vi "Barker7.vi"(9 "Barker code":i16[](array[numeric])=[16384, 16384, 16384, -16384, -16384, 16384, -16384], 10 "Barker width":u16, 11 "first?":bool) -> (2 "output":i16, 3 "output valid":bool)   [LabVIEW 2017]
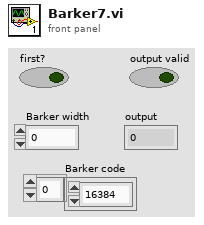
[diagram p1: front panel]
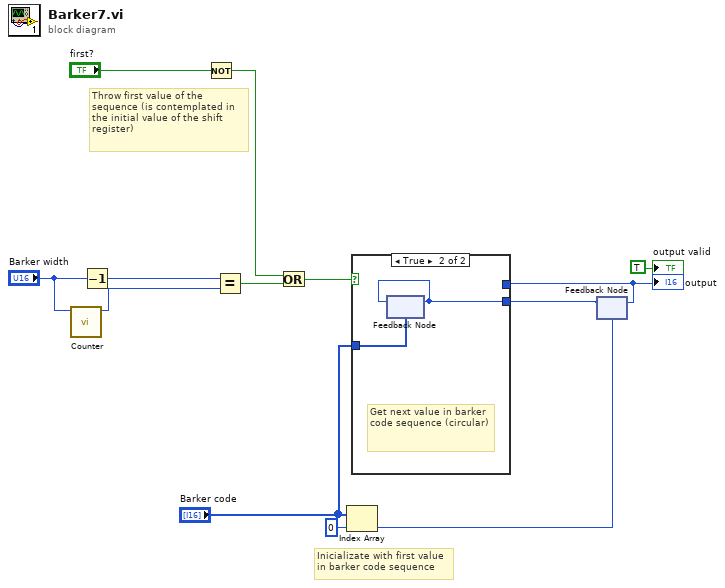
[diagram p0: block diagram]
diagram:
  # "Throw first value of the sequence (is contemplated in the initial value of the shift register)"
  # "Inicializate with first value in barker code sequence"
  n1 = call "Counter.vi"("limit"="Barker width") -> ("count"=w12:u32)  [unwired: 9 in, 1 out]
  n2 = Decrement(x="Barker width") -> (x-1=w3:u16)
  n3 = Not(x="first?") -> (.not. x?=w5:bool)
  n4 = Equal?(x=w3, y=w12) -> (x = y?=w6:bool)
  n5 = Or(x=w5, y=w6) -> (x .or. y?=w7:bool)
  n6 = Index Array(array="Barker code", index=0) -> (element=w2:i16)
  n7 = feedback #1(w2) -> (w10:i16)
  "output" <- w10
  n8 = case shown="True" w7 {
    tunnel: [w14 w15] -> w4
    tunnel: "Barker code" -> [_ w16]
    tunnel: w10 -> [w14 _]
    frame False {
      # "Get last value used in barker code sequence"
    }
    frame True {
      # "Get next value in barker code sequence (circular)"
      n9 = feedback #2(w16) -> (w15:i16)
      n10 = feedback-in #2(w15) -> ()
    }
  }
  n11 = feedback-in #1(w4) -> ()
  "output valid" <- TRUE ("output valid")
